vi "write single register.vi"(8 "error in (no error)":errorcluster, 9 "register to write":u16 format="%.0x", 10 "address":u16 format="%.0x", 11 "CL57RS in":refnum<class "CL57RS.lvclass">) -> (0 "error out":errorcluster, 3 "CL57RS out":refnum<class "CL57RS.lvclass">)   [LabVIEW 2025, in "Motor.lvlib" / "CL57RS.lvclass"]
uses:
  CL57RS.lvclass
  CL57RS.lvclass/CL57RS.ctl
  <vilib>/NI/Modbus Library/API/Master/Modbus Master.lvclass
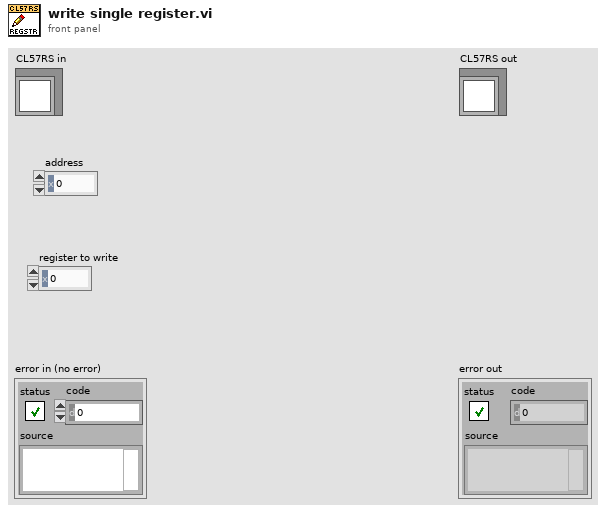
[diagram p1: front panel]
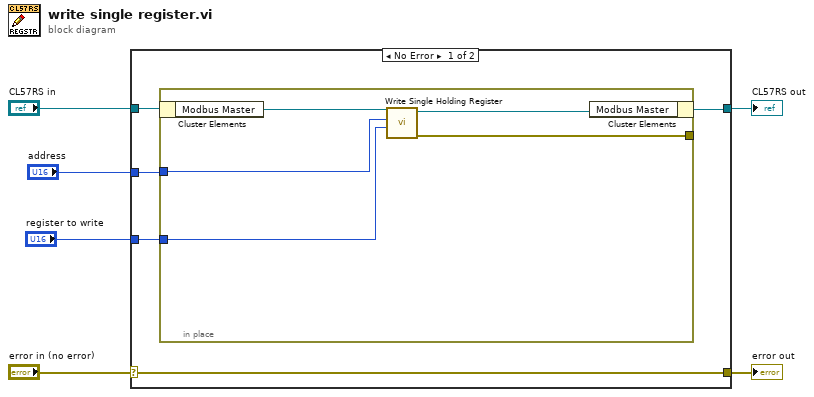
[diagram p0: block diagram]
diagram:
  n1 = case shown="No Error" "error in (no error)" {
    selector: "error in (no error)" -> [w11 w18]
    tunnel: [w11 w18] -> w5
    tunnel: [w9 w17] -> w3
    tunnel: "CL57RS in" -> [w10 w17]
    tunnel: "register to write" -> [w8 _]
    tunnel: "address" -> [w7 _]
    frame No Error {
      n2 = in-place {
        in-place-border: w7 -> [w14]
        in-place-border: w8 -> [w13]
        in-place-border: [w12] -> _
        n3 = in-place-cluster #1(w10) -> ("Modbus Master"=w16:refnum<class "Modbus Master.lvclass">)
        n4 = call-dynamic "Write Single Holding Register.vi"("register to write"=w13, "address"=w14, "Modbus master in"=w16) -> ("error out"=w12:errorcluster, "Modbus master out"=w15:refnum<class "Modbus Master.lvclass">)  [unwired: 7 in]
        n5 = in-place-cluster #1("Modbus Master"=w15) -> (w9:refnum<class "CL57RS.lvclass">)
      }
    }
    frame Error {
    }
  }
  "error out" <- w5
  "CL57RS out" <- w3
